vi "Principle Eigenpair.vi"(10 "Matrix":T1) -> (2 "Principal Eigenvector":dbl[](array[numeric]), 3 "Principle Eigenvalue":dbl)   [LabVIEW 2011]
uses:
  <vilib>/Analysis/Matrix/Datatypes/RealMatrix.ctl
  <vilib>/Analysis/7linalg.llb/Real Eigenvalues and Vectors.vi
  <vilib>/Analysis/Matrix/Numeric/Complex/Complex To Cartesian - CM.vi
  <vilib>/Analysis/NI_AALPro.lvlib
  <vilib>/Analysis/Matrix/NI_Matrix.lvlib
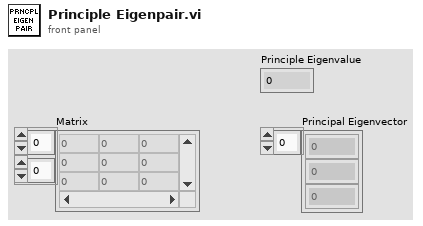
[diagram p1: front panel]
types:
  T1 = typedef "NI_Matrix.lvlib/RealMatrix.ctl" = dbl[][]
  T2 = typedef "NI_Matrix.lvlib/ComplexMatrix.ctl" = cdb[][]
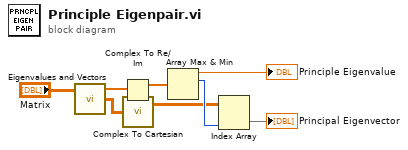
[diagram p0: block diagram]
diagram:
  n1 = call-poly <vilib>:"Eigenvalues and Vectors.vi"("Input Matrix"="Matrix") -> ("Eigenvectors"=w3:T2, "Eigenvalues"=w7:cdb[])  [unwired: 2 in, 1 out]
  n2 = Complex To Re/Im(x + iy=w7) -> (x=w6:dbl[])  [unwired: 1 out]
  n3 = call-poly <vilib>:"Complex To Cartesian.vi"("Complex Matrix R + Ii"=w3) -> ("Real Matrix R"=w2:T1)  [unwired: 1 out]
  n4 = Array Max & Min(array=w6) -> (max value=→"Principle Eigenvalue":dbl, max index (indices)=w5:i32)  [unwired: 2 out]
  n5 = Index Array(array=w2, index (col)=w5) -> (element=→"Principal Eigenvector":dbl[])  [unwired: 1 in]
